vi "operate.vi"(0 "reference in":refnum<class "Master Controller.lvclass">, 5 "error in (no error)":errorcluster) -> (14 "reference out":refnum<class "Master Controller.lvclass">, 19 "error out":errorcluster)   [LabVIEW 2015, in "Master Controller.lvclass"]
uses:
  Master Controller.lvclass
  GUI/GUI Controller_llb/GUI Controller.lvclass
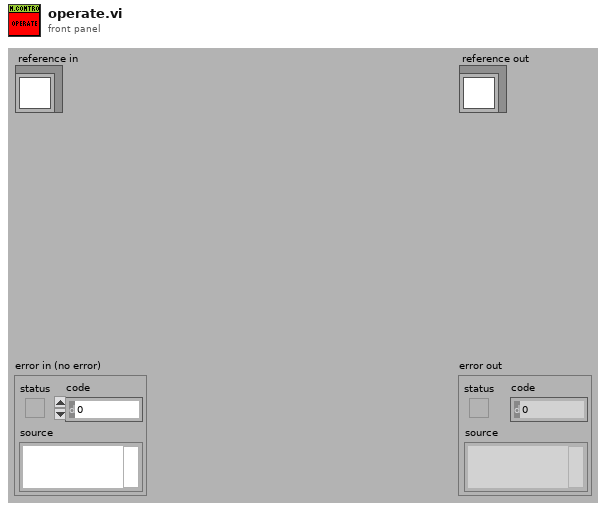
[diagram p1: front panel]
types:
  T1 = typedef "Master Controller.lvclass/ObjectAttributesRef.ctl" = refnum<data-value>
  T2 = typedef "Master Controller.lvclass/ObjectAttributes.ctl" = cluster{"MyAttribute":dbl, "Devices Controller_ref":refnum<class "Devices Controller.lvclass">, "File Controller_ref":refnum<class "File Controller.lvclass">, "Items Controller_ref":refnum<class "Items Controller.lvclass">, "GUI Controller_ref":refnum<class "GUI Controller.lvclass">, "NotificationController_ref":refnum<class "Notification Controller.lvclass">, "PartsTracking Controller_ref":refnum<class "PartsTracking Controller.lvclass">}
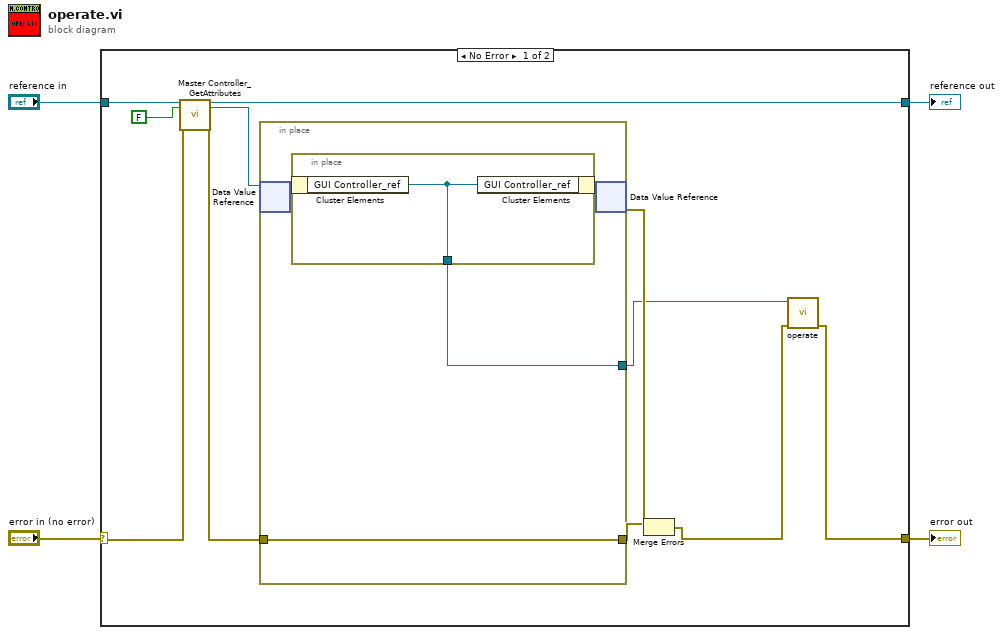
[diagram p0: block diagram]
diagram:
  n1 = case shown="No Error" "error in (no error)" {
    selector: "error in (no error)" -> [w11 w22]
    tunnel: [w5 w22] -> w3
    tunnel: [w9 w21] -> w1
    tunnel: "reference in" -> [w13 w21]
    frame No Error {
      n2 = call "Master Controller_GetAttributes.vi"("reference in"=w13, "return data? (T)"=FALSE, "error in (no error)"=w11) -> ("reference out"=w9:refnum<class "Master Controller.lvclass">, "attributes ref"=w8:T1, "error out"=w10:errorcluster)  [unwired: 13 in, 1 out]
      n3 = in-place {
        in-place-border: w10 -> [w17]
        in-place-border: [w17] -> w14
        in-place-border: [w16] -> w7
        n4 = in-place-dvr #1(w8) -> (w18:T2)  [unwired: 1 out]
        n5 = in-place {
          in-place-border: [w20] -> w16
          n6 = in-place-cluster #2(w18) -> ("GUI Controller_ref"=w20:refnum<class "GUI Controller.lvclass">)
          n7 = in-place-cluster #2("GUI Controller_ref"=w20) -> (w19:T2)
        }
        n8 = in-place-dvr #1(w19) -> (w15:errorcluster)  [unwired: 1 out]
      }
      n9 = Merge Errors(w14, w15) -> (w6:errorcluster)
      n10 = call "operate.vi"("error in (no error)"=w6, "reference in"=w7) -> ("error out"=w5:errorcluster)  [unwired: 8 in, 1 out]
    }
    frame Error {
    }
  }
  "error out" <- w3
  "reference out" <- w1
